vi "Close.vi"(8 "error in (no error)":errorcluster, 11 "Facade in":refnum<class "Facade.lvclass">) -> (0 "error out":errorcluster, 2 "ProcessMessage":string, 3 "Facade out":refnum<class "Facade.lvclass">)   [LabVIEW 2013, in "Facade.lvclass"]
uses:
  Facade.lvclass
  Facade.lvclass/Facade.ctl
  RoomLight.lvclass/RoomLight.lvclass
  CDPlayer.lvclass/CDPlayer.lvclass
  DVDPlayer.lvclass/DVDPlayer.lvclass
  Projector.lvclass/Projector.lvclass
  Tuner.lvclass/Tuner.lvclass
  Amplifer.lvclass/Amplifer.lvclass
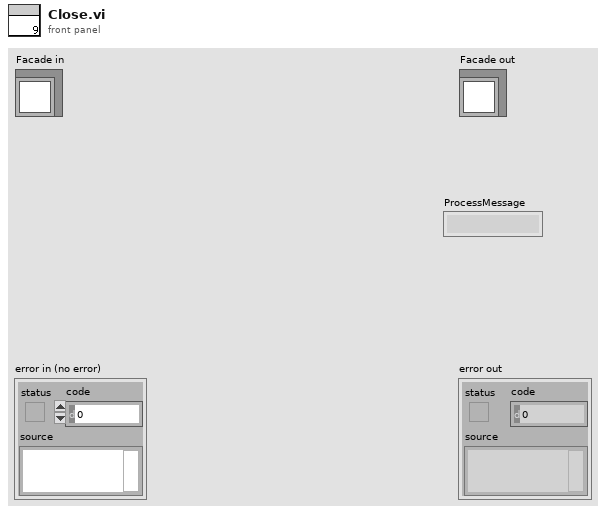
[diagram p1: front panel]
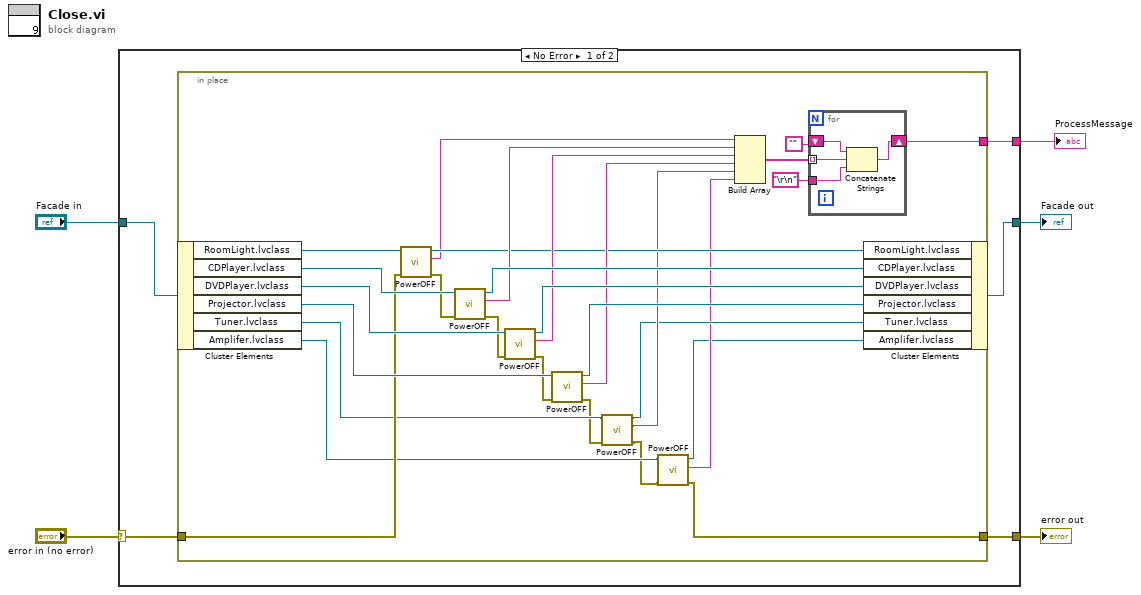
[diagram p0: block diagram]
diagram:
  n1 = case shown="No Error" "error in (no error)" {
    selector: "error in (no error)" -> [w10 w45]
    tunnel: [w6 w45] -> w4
    tunnel: [w8 w44] -> w2
    tunnel: "Facade in" -> [w9 w44]
    tunnel: [w7 _] -> w1
    frame No Error {
      n2 = in-place {
        in-place-border: w10 -> [w20]
        in-place-border: [w36] -> w7
        in-place-border: [w13] -> w6
        n3 = in-place-cluster #1(w9) -> ("RoomLight.lvclass"=w24:refnum<class "RoomLight.lvclass">, "CDPlayer.lvclass"=w35:refnum<class "CDPlayer.lvclass">, "DVDPlayer.lvclass"=w34:refnum<class "DVDPlayer.lvclass">, "Projector.lvclass"=w33:refnum<class "Projector.lvclass">, "Tuner.lvclass"=w19:refnum<class "Tuner.lvclass">, "Amplifer.lvclass"=w15:refnum<class "Amplifer.lvclass">)
        n4 = call-dynamic "PowerOFF.vi"("error in (no error)"=w20, "RoomLight in"=w24) -> ("error out"=w21:errorcluster, "Message"=w22:string, "RoomLight out"=w23:refnum<class "RoomLight.lvclass">)  [unwired: 7 in]
        n5 = call-dynamic "PowerOFF.vi"("error in (no error)"=w21, "CDPlayer in"=w35) -> ("error out"=w32:errorcluster, "Message"=w27:string, "CDPlayer out"=w30:refnum<class "CDPlayer.lvclass">)  [unwired: 7 in]
        n6 = call-dynamic "PowerOFF.vi"("error in (no error)"=w32, "DVDPlayer in"=w34) -> ("error out"=w31:errorcluster, "Message"=w26:string, "DVDPlayer out"=w29:refnum<class "DVDPlayer.lvclass">)  [unwired: 7 in]
        n7 = call-dynamic "PowerOFF.vi"("error in (no error)"=w31, "Projector in"=w33) -> ("error out"=w18:errorcluster, "Message"=w25:string, "Projector out"=w28:refnum<class "Projector.lvclass">)  [unwired: 7 in]
        n8 = call-dynamic "PowerOFF.vi"("error in (no error)"=w18, "Tuner in"=w19) -> ("error out"=w14:errorcluster, "Message"=w17:string, "Tuner out"=w16:refnum<class "Tuner.lvclass">)  [unwired: 7 in]
        n9 = call-dynamic "PowerOFF.vi"("error in (no error)"=w14, "Amplifer in"=w15) -> ("error out"=w13:errorcluster, "Message"=w12:string, "Amplifer out"=w11:refnum<class "Amplifer.lvclass">)  [unwired: 7 in]
        n10 = Build Array(w22, w27, w26, w25, w17, w12) -> (w39:string[])
        n11 = for {
          tunnel: w39 -> [w40] mode=indexing
          tunnel: "\r\n" -> [w43]
          shift-right: [w41] -> w36
          shift-left: "" -> [w42]
          n12 = Concatenate Strings(w42, w40, w43) -> (w41:string)
        }
        n13 = in-place-cluster #1("RoomLight.lvclass"=w23, "CDPlayer.lvclass"=w30, "DVDPlayer.lvclass"=w29, "Projector.lvclass"=w28, "Tuner.lvclass"=w16, "Amplifer.lvclass"=w11) -> (w8:refnum<class "Facade.lvclass">)
      }
    }
    frame Error {
    }
  }
  "error out" <- w4
  "Facade out" <- w2
  "ProcessMessage" <- w1
